vi "ICA_10_Potluri.vi"() -> ()   [LabVIEW 2016]
uses:
  <vilib>/NXT/Subs/LVHSConnector.ctl
  <vilib>/NXT/LegoClasses/BrickReference/BrickReference.lvclass
  <vilib>/NXT/Block Support/NXT_InputPort.ctl
  <vilib>/NXT/Dual Mode Library/Sensors/EV3_Color_RGB.vi
  <vilib>/NXT/Dual Mode Library/Sensors/EV3_Ultrasonic_IN.vi
panel:
  out "NXT/EV3 4":T1
  out "Centimeters":sgl
  in  "Port (Port 1) 2":T2 items=["Port 1", "Port 2", "Port 3", "Port 4"]
  in  "NXT/EV3 3":T1
  out "RGB Color":cluster{"Red":u8, "Green":u8, "Blue":u8}
  out "NXT/EV3 2":T1
  in  "Port (Port 1)":T2 items=["Port 1", "Port 2", "Port 3", "Port 4"]
  in  "NXT/EV3":T1
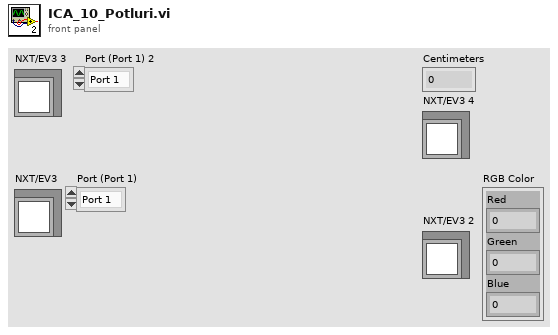
[diagram p1: front panel]
types:
  T1 = typedef "LVHSConnector.ctl" = refnum<class "BrickReference.lvclass">
  T2 = typedef "NXT_InputPort.ctl" = u32
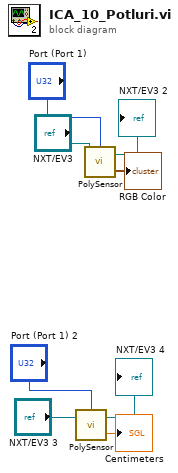
[diagram p0: block diagram]
diagram:
  n1 = call-poly <vilib>:"PolySensor.vi"("NXT/EV3"="NXT/EV3 3", "Port (Port 1)"="Port (Port 1) 2") -> ("Inches"=→"Centimeters":sgl, "NXT/EV3"=→"NXT/EV3 4":T1)  [unwired: 1 in]
  n2 = call-poly <vilib>:"PolySensor.vi"("NXT/EV3"="NXT/EV3", "Port (Port 1)"="Port (Port 1)") -> ("RGB Color"=→"RGB Color":cluster{"Red":u8, "Green":u8, "Blue":u8}, "NXT/EV3"=→"NXT/EV3 2":T1)  [unwired: 1 in]
